vi "Float Decoder.vi"(7 "Optional":bool, 8 "error in (no error)":errorcluster, 9 "Array":u8[](array[numeric]) format="%02x", 10 "Key":i32=-1) -> (0 "error out":errorcluster, 1 "array w/ subset deleted":u8[](array[numeric]), 2 "Read Key":i32, 3 "Float":sgl)   [LabVIEW 2020]
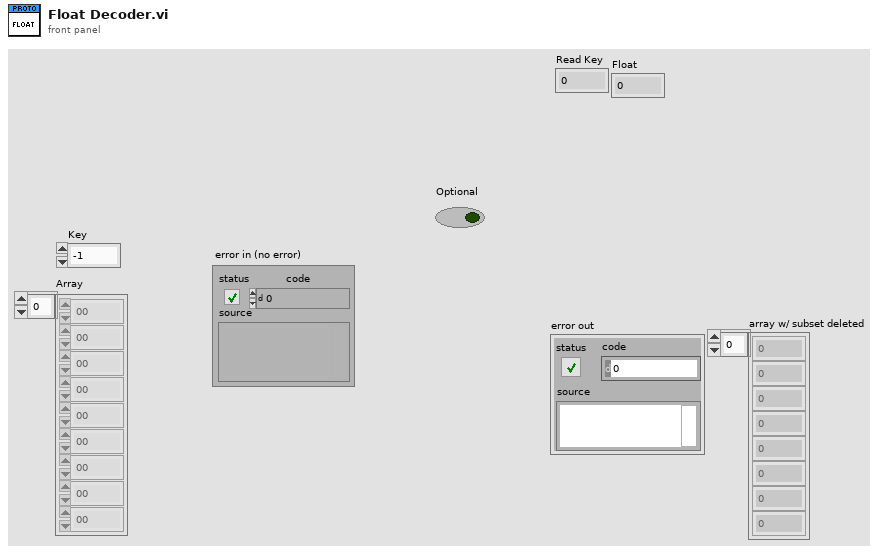
[diagram p1: front panel]
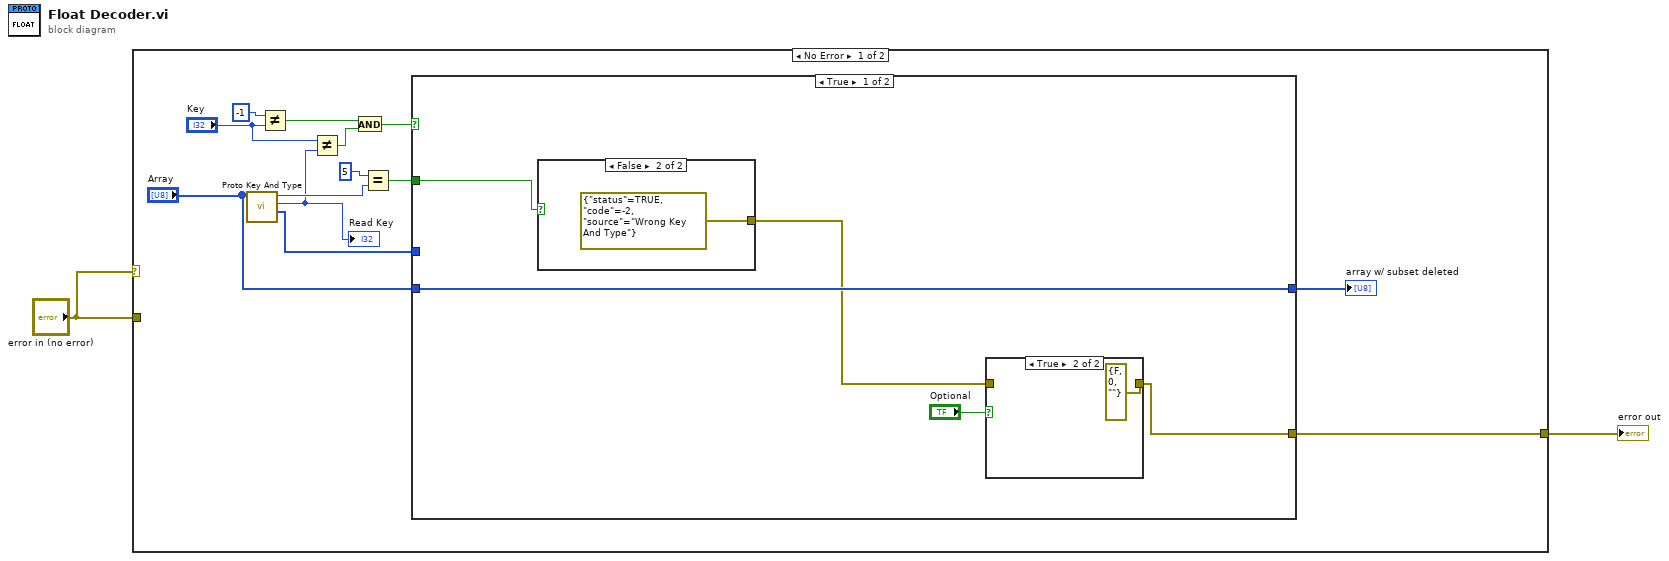
[diagram p0: block diagram]
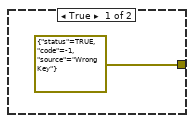
[diagram p3: hidden frame]
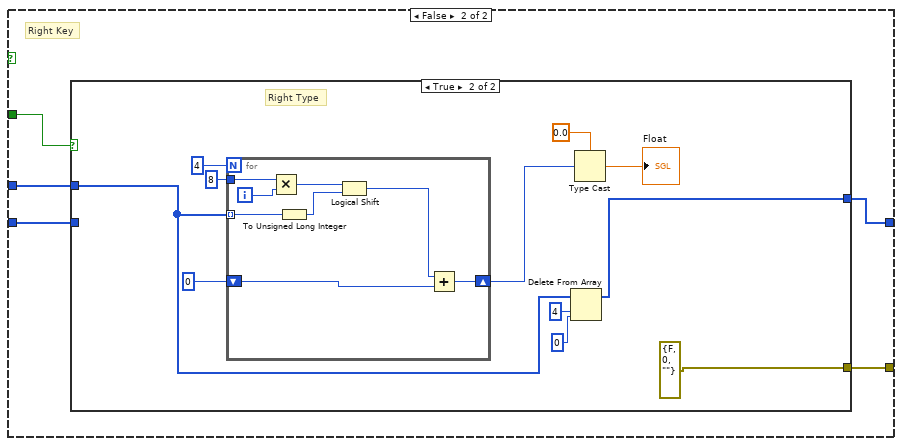
[diagram p4: hidden frame]
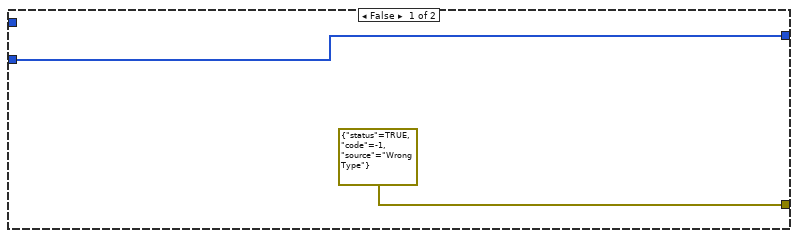
[diagram p5: hidden frame]
diagram:
  n1 = case shown="No Error" "error in (no error)" {
    tunnel: "error in (no error)" -> [_ w51]
    tunnel: [w3 w51] -> w1
    frame No Error {
      n2 = call "Proto Key And Type.vi"("Array"="Array") -> ("array w/ subset deleted"=w15:u8[], "Key"=w4:i32, "Type"=w7:i32)  [unwired: 8 in]
      "Read Key" <- w4
      n3 = Not Equal?(x=-1, y="Key") -> (x != y?=w12:bool)
      n4 = Not Equal?(x="Key", y=w4) -> (x != y?=w10:bool)
      n5 = And(x=w12, y=w10) -> (x .and. y?=w9:bool)
      n6 = Equal?(x=5, y=w7) -> (x = y?=w6:bool)
      n7 = case shown="True" w9 {
        tunnel: w15 -> [_ w29]
        tunnel: "Array" -> [w19 w28]
        tunnel: w6 -> [w20 w27]
        tunnel: [w16 w26] -> w3
        tunnel: [w19 w25] -> w5
        frame True {
          n8 = case shown="False" w20 {
            tunnel: [errorcluster {"status"=TRUE, "code"=-1, "source"="Wrong Key"} ("error in (no error)") errorcluster {"status"=TRUE, "code"=-2, "source"="Wrong Key And Type"} ("error in (no error)")] -> w17
            frame True {
            }
            frame False {
            }
          }
          n9 = case shown="True" "Optional" {
            tunnel: w17 -> [w21 _]
            tunnel: [w21 errorcluster {"status"=FALSE, "code"=0, "source"=""} ("error in (no error)")] -> w16
            frame False {
            }
            frame True {
            }
          }
        }
        frame False {
          # "Right Key"
          n10 = case shown="True" w27 {
            tunnel: [errorcluster {"status"=TRUE, "code"=-1, "source"="Wrong Type"} ("error in (no error)") errorcluster {"status"=FALSE, "code"=0, "source"=""} ("error in (no error)")] -> w26
            tunnel: w29 -> [_ w39]
            tunnel: [w30 w38] -> w25
            tunnel: w28 -> [w30 _]
            frame False {
            }
            frame True {
              # "Right Type"
              n11 = for {
                N: 4 -> [_]
                tunnel: w39 -> [w44] mode=indexing
                shift-right: [w50] -> w35
                shift-left: u32 0 -> [w45]
                tunnel: 8 -> [w48]
                i -> [w49]
                n12 = Multiply(x=w48, y=w49) -> (x*y=w47:i32)
                n13 = To Unsigned Long Integer(number=w44) -> (unsigned 32bit integer=w43:u32)
                n14 = Logical Shift(y=w47, x=w43) -> (x << y=w46:u32)
                n15 = Add(x=w46, y=w45) -> (x+y=w50:u32)
              }
              n16 = Delete From Array(array=w39, length=4, index=0) -> (array with subset deleted=w38:u8[])  [unwired: 1 out]
              n17 = Type Cast(type=sgl 0.0, x=w35) -> (*(type *) &x=→"Float":sgl)
            }
          }
        }
      }
      "array w/ subset deleted" <- w5
    }
    frame Error {
    }
  }
  "error out" <- w1
